vi "Cam0 AprilTag Target Package.vi"(0 "Camera Name":string="cam0") -> ()   [LabVIEW 2023]
uses:
  <vilib>/vision/Shape Detection.llb/ShapeDetectionMatchOptions.ctl
  <vilib>/vision/Pattern Matching.llb/IMAQ Match Range Setting.ctl
  <vilib>/vision/Image Controls.llb/IMAQ Image.ctl
  Camera Set Up/Event Setup Types.ctl
  <vilib>/Utility/config.llb/Write Key (String).vi
  <vilib>/Utility/config.llb/Read Key (String).vi
  <vilib>/Utility/config.llb/NI_LVConfig.lvlib
  <vilib>/vision/NI_Vision_Development_Module.lvlib
panel:
  in  "Main":enum32{"Page 1", "Page 2"}(tab)
  out "Image":T1(plugin-control)
  in  "Settings":bool
  in  "Save":bool
  in  "Tools":bool
  in  "Min Level":dbl=40.0 format="%#_13g"
  out "Fps":dbl format="%#.0f"
  in  "Target Size":dbl=6.5
  out "Distance":dbl[](array[numeric]) format="%.1f"
  out "Angle":dbl[](array[numeric]) format="%.1f"
  in  "Min Rectangle Size (pix)":dbl
  in  "Max Rectangle Size (pix)":dbl
  in  "Home":bool
  in  "Match Options":T2={"Rotation"=TRUE, "Scale"=TRUE, "Occlusion"=FALSE, "Range Settings"=[]} {"Range Settings"."Match Constraints" items=["Rotation Angle (degrees)", "Scale Factor (%)", "Occlusion (%)"]}
  in  "upper limit":sgl=1.2
  in  "lower limit":sgl=0.8
  # "Aspect Ratio"
  # "Range"
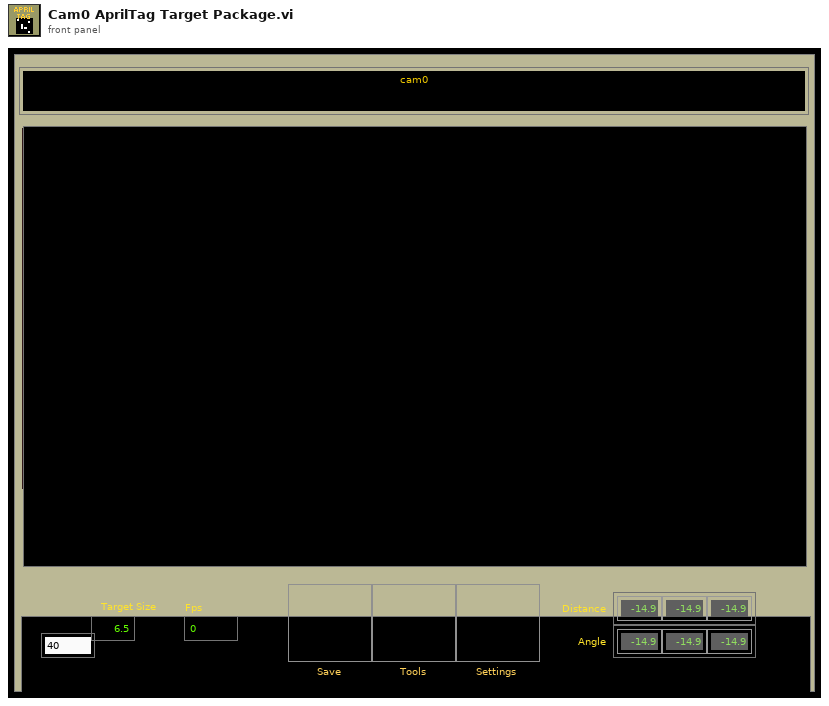
[diagram p1: front panel]
types:
  T1 = typedef "IMAQ Image.ctl" = refnum<image>
  T2 = typedef "ShapeDetectionMatchOptions.ctl" = cluster{"Rotation":bool, "Scale":bool, "Occlusion":bool, "Range Settings":T3[]}
  T3 = typedef "IMAQ Match Range Setting.ctl" = cluster{"Match Constraints":u32, "Min":dbl, "Max":dbl}
  T4 = typedef "Image Type" = u32
  T5 = cluster{"Min Width":dbl, "Max Width":dbl, "Min Height":dbl, "Max Height":dbl}
  T6 = typedef "Event Setup Types.ctl" = enum16{"Default", "Camera Loop Started", "Save Data", "Open Front Panel", "Exit"}
  T7 = cluster{"Corners":cluster{"X":sgl, "Y":sgl}[], "Angle":dbl, "Width":dbl, "Height":dbl, "Score":dbl}[]
  T8 = typedef "Target Fields.ctl" = cluster{"diameter points":cluster{"first point":cluster{"x":dbl, "y":dbl}, "projected point":cluster{"x":dbl, "y":dbl}}, "normalized center":cluster{"x":dbl, "y":dbl}, "Overall Score":dbl, "Area Score":dbl, "Moment Score":dbl, "Aspect Score":dbl, "Distance (ft)":dbl, "Upper Goal":bool}
  T9 = typedef "NI_LVConfig.lvlib/Config Data RefNum.ctl" = refnum<k1>
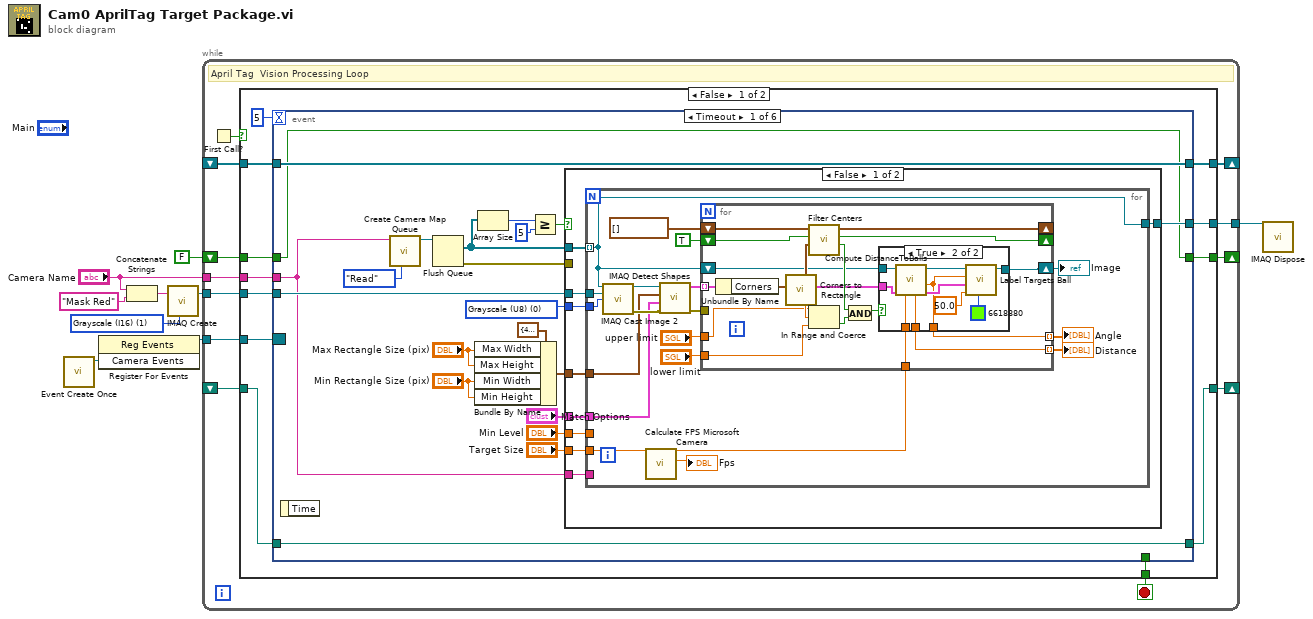
[diagram p0: block diagram]
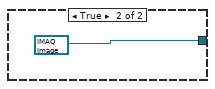
[diagram p3: hidden frame]
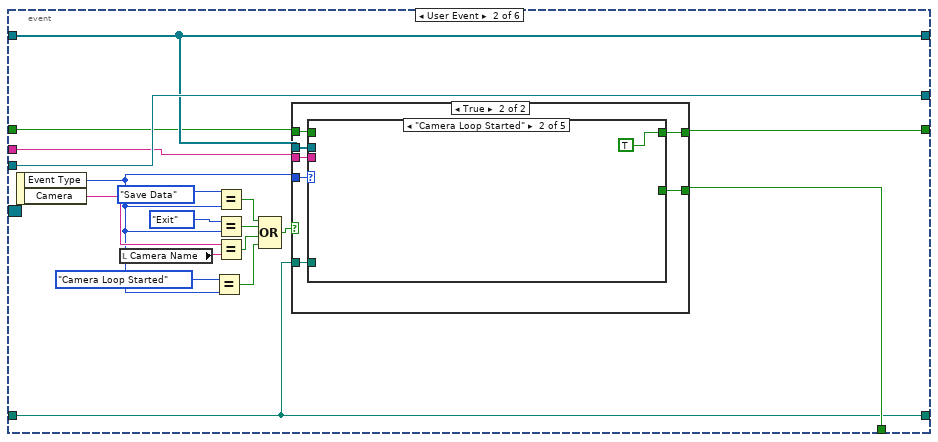
[diagram p4: hidden frame]
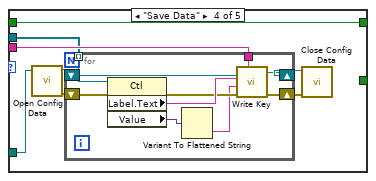
[diagram p8: hidden frame]
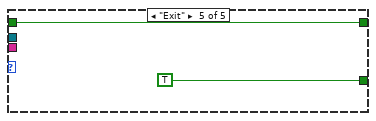
[diagram p9: hidden frame]
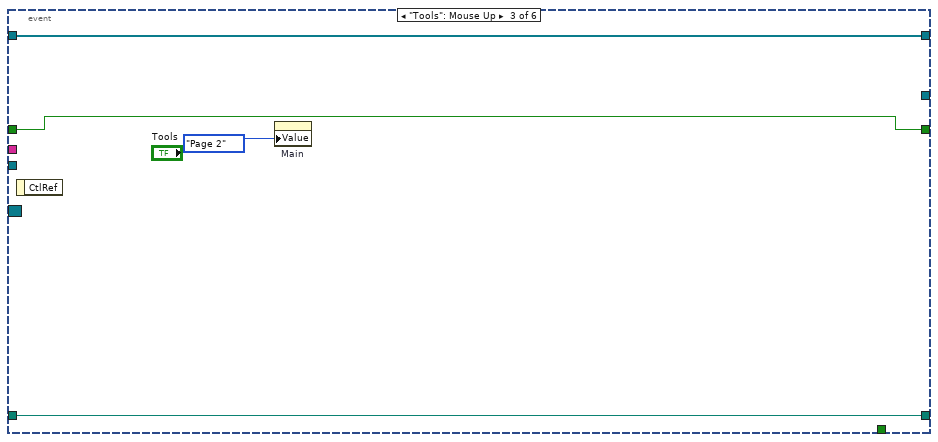
[diagram p10: hidden frame]
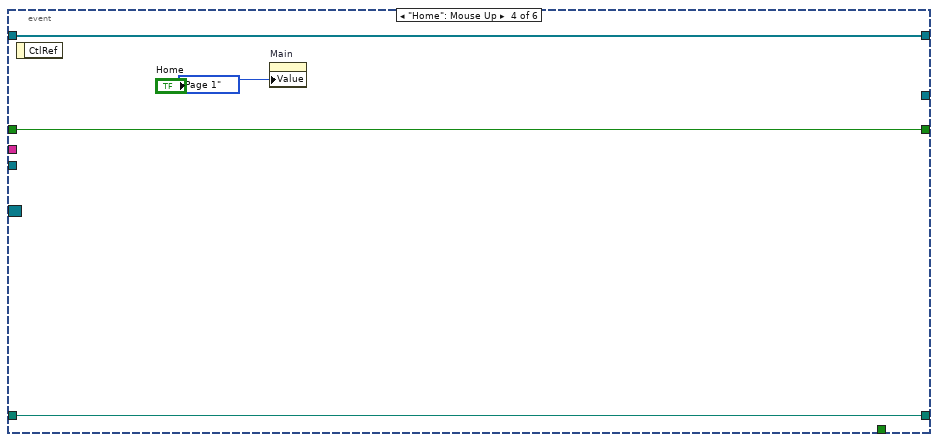
[diagram p11: hidden frame]
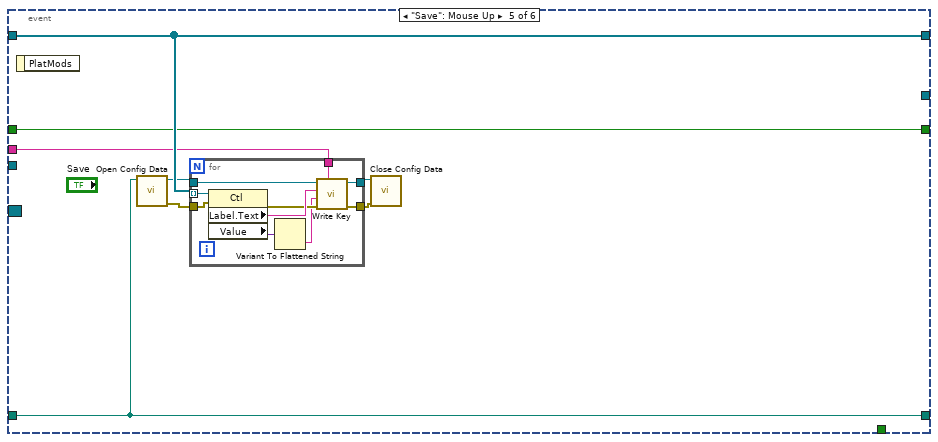
[diagram p12: hidden frame]
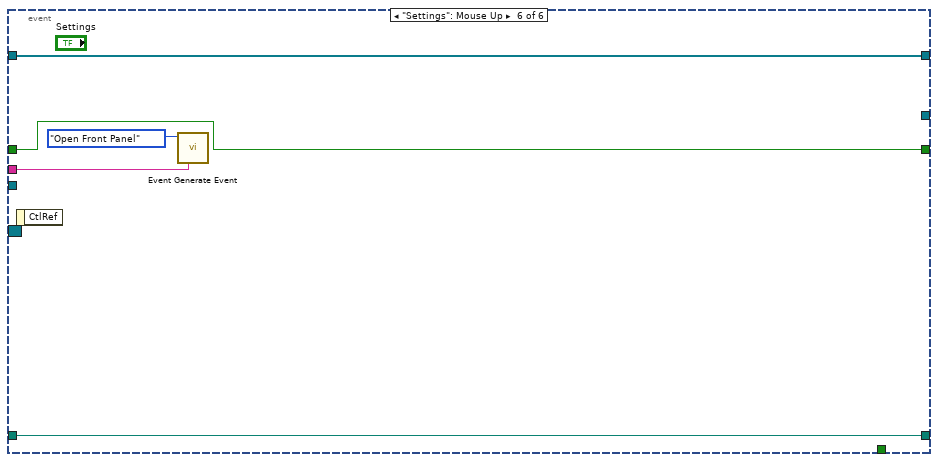
[diagram p13: hidden frame]
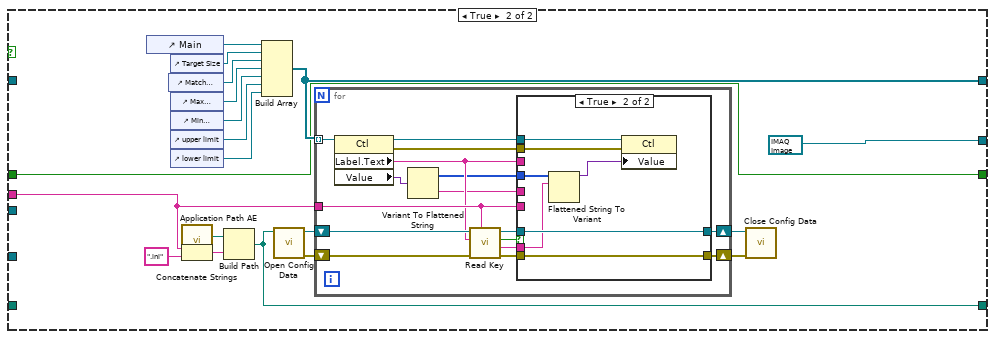
[diagram p14: hidden frame]
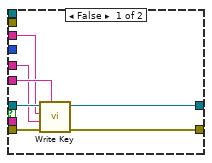
[diagram p15: hidden frame]
diagram:
  w6 = T4 1 items=["Grayscale (U8)", "Grayscale (I16)", "Grayscale (SGL)", "Complex (CSG)", "RGB (U32)", "HSL (U32)", "RGB (U64)", "Grayscale (U16)"] ("Image Type")
  n1 = call "Event Create Once.vi"() -> ("Camera Events"=w8:refnum<user-event>)  [unwired: 10 in, 1 out]
  n2 = register-events(w8) -> (reference out=w7:refnum<event-registration>)  [unwired: 2 in, 1 out]
  n3 = Concatenate Strings("Camera Name", "Mask Red" ("string")) -> (w5:string)
  n4 = call "IMAQ Create"("Image Name"=w5, "Image Type"=w6) -> ("New Image"=w9:T1)  [unwired: 2 in, 2 out]
  n5 = while {
    tunnel: w9 -> [w21]
    tunnel: [w20] -> w1
    tunnel: w7 -> [w19]
    tunnel: "Camera Name" -> [w17]
    shift-right: [w15] -> _
    shift-left: _ -> [w14]
    shift-right: [w13] -> _
    shift-left: _ -> [w12]
    shift-right: [w10] -> _
    shift-left: FALSE -> [w11]
    stop <- w18 stop-if-true
    # "April Tag  Vision Processing Loop"
    n6 = First Call?() -> (First Call?: T/F=w16:bool)
    n7 = case shown="False" w16 {
      tunnel: w21 -> [w33 _]
      tunnel: [w32 T1 refnum ("New Image")] -> w20
      tunnel: w19 -> [w31 _]
      tunnel: [w30 _] -> w18
      tunnel: w17 -> [w29 w205]
      tunnel: [w27 w201] -> w15
      tunnel: w14 -> [w28 _]
      tunnel: [w26 w204] -> w13
      tunnel: w12 -> [w24 _]
      tunnel: w11 -> [w23 w198]
      tunnel: [w22 w198] -> w10
      frame False {
        n8 = event shown="[0] Timeout" {
          selector: w31 -> [_ _ _ _ _ _]
          dyn-events: _ -> [_ _ _ _ _ _]
          timeout: 5 -> [_ _ _ _ _ _]
          tunnel: w33 -> [w53 w130 _ _ _ _]
          tunnel: [w54 w130 _ _ _ _] -> w32
          tunnel: [_ w129 _ _ _ _] -> w30
          tunnel: w29 -> [w50 w128 _ _ w173 w189]
          tunnel: w28 -> [w52 w126 w165 w169 w176 w192]
          tunnel: [w52 w126 w165 w169 w176 w192] -> w27
          tunnel: w24 -> [w51 w127 w164 w168 w177 w191]
          tunnel: [w51 w127 w164 w168 w177 w191] -> w26
          tunnel: w23 -> [w49 w117 w162 w166 w170 w188]
          tunnel: [w49 w116 w162 w166 w170 w188] -> w22
          event Timeout {
            w44 = T4 0 items=["Grayscale (U8)", "Grayscale (I16)", "Grayscale (SGL)", "Complex (CSG)", "RGB (U32)", "HSL (U32)", "RGB (U64)", "Grayscale (U16)"] ("Image Type")
            n9 = event-data() -> ()  [unwired: 1 in, 1 out]
            n10 = call "Create Camera Map Queue.vi"("Action"=enum16{"Read", "Write"}."Read", "Camera"=w50) -> ("value"=w46:refnum<queue>)  [unwired: 8 in, 1 out]
            n11 = Flush Queue(queue=w46) -> (remaining elements=w43:T1[], error out=w45:errorcluster)  [unwired: 1 in, 1 out]
            n12 = Bundle By Name(cluster=T5 {"Min Width"=40.0, "Max Width"=100.0, "Min Height"=40.0, "Max Height"=200.0} ("Rectangle Descriptor"), "Max Width"="Max Rectangle Size (pix)", "Max Height"="Max Rectangle Size (pix)", "Min Width"="Min Rectangle Size (pix)", "Min Height"="Min Rectangle Size (pix)") -> (w36:T5)
            n13 = Array Size(array=w43) -> (size(s)=w42:i32)
            n14 = Greater Or Equal?(x=w42, y=5) -> (x >= y?=w40:bool)
            n15 = case shown="False" w40 {
              tunnel: [w55 T1 refnum ("Image")] -> w54
              tunnel: w53 -> [w63 _]
              tunnel: w50 -> [w62 _]
              tunnel: "Target Size" -> [w61 _]
              tunnel: w43 -> [w60 _]
              tunnel: w45 -> [_ _]
              tunnel: w44 -> [w59 _]
              tunnel: "Min Level" -> [w58 _]
              tunnel: w36 -> [w57 _]
              tunnel: "Match Options" -> [w56 _]
              frame False {
                n16 = for {
                  tunnel: w63 -> [w81]
                  tunnel: w60 -> [w70] mode=indexing
                  tunnel: w62 -> [_]
                  tunnel: w61 -> [w69]
                  tunnel: w59 -> [w80]
                  tunnel: w58 -> [_]
                  tunnel: w57 -> [w76]
                  tunnel: w56 -> [w75]
                  tunnel: [w70] -> w55
                  n17 = call "IMAQ Cast Image 2"("Image Src"=w70, "Image Dst"=w81, "Image Type"=w80) -> ("Image Dst Out"=w78:T1, "error out"=w77:errorcluster)  [unwired: 11 in]
                  n18 = call "Calculate FPS Microsoft Camera.vi"() -> ("Fps"=→"Fps":dbl)  [unwired: 11 in]
                  n19 = call-poly "IMAQ Detect Shapes"("error in (no error)"=w77, "Match Options"=w75, "Rectangle Descriptor"=w76, "Image"=w78) -> ("error out"=w66:errorcluster, "Rectangles"=w72:T7)  [unwired: 5 in, 1 out]
                  n20 = for {
                    shift-right: [w82] -> w71
                    shift-left: w70 -> [w83]
                    shift-right: [w97] -> _
                    shift-left: cluster{"X":dbl, "Y":dbl}[] [] ("Centers 2") -> [w99]
                    shift-right: [w95] -> _
                    shift-left: TRUE -> [w96]
                    tunnel: w72 -> [w91] mode=indexing
                    tunnel: w69 -> [w88]
                    tunnel: [w87] -> w67 mode=indexing
                    tunnel: [w86] -> w68 mode=indexing
                    tunnel: w66 -> [_]
                    tunnel: "lower limit" -> [w85]
                    tunnel: "upper limit" -> [w84]
                    n21 = Unbundle By Name(w91) -> ("Corners"=w90:cluster{"X":sgl, "Y":sgl}[])
                    n22 = call "Corners to Rectangle.vi"("Corners 2"=w90) -> ("output cluster"=w89:T8, "Aspect Ratio"=w100:sgl, "Center"=w98:cluster{"X":dbl, "Y":dbl})  [unwired: 8 in]
                    n23 = call "Filter Centers.vi"("Center"=w98, "First time"=w96, "Centers"=w99) -> ("Added"=w94:bool, "First time Out"=w95:bool, "Centers 2"=w97:cluster{"X":dbl, "Y":dbl}[])  [unwired: 6 in]
                    n24 = In Range and Coerce(upper limit=w84, x=w100, lower limit=w85) -> (In Range?=w93:bool)  [unwired: 1 out]
                    n25 = And(x=w94, y=w93) -> (x .and. y?=w92:bool)
                    n26 = case shown="True" w92 {
                      tunnel: w83 -> [w101 w110]
                      tunnel: [w101 w111] -> w82
                      tunnel: w89 -> [_ w105]
                      tunnel: w88 -> [_ w104]
                      tunnel: [_ w103] -> w87
                      tunnel: [_ w102] -> w86
                      frame False {
                      }
                      frame True {
                        n27 = call "Compute DistanceToBalls.vi"("Target Width (in)"=w104, "results"=w105, "Image Src"=w110) -> ("results out"=w106:T8, "Off Angle"=w102:dbl, "Image Dst Out"=w108:T1, "Distance"=w103:dbl)  [unwired: 4 in, 1 out]
                        n28 = call "Label Targets Ball.vi"("Color"=u32 6618880, "Score Threshold"=50.0, "results"=w106, "Angle"=w102, "Image in"=w108) -> ("Image out"=w111:T1)  [unwired: 6 in]
                      }
                    }
                  }
                  "Image" <- w71
                  "Angle" <- w68
                  "Distance" <- w67
                }
              }
              frame True {
              }
            }
          }
          event User Event {
            n29 = event-data() -> ("Event Type"=w115:T6, "Camera"=w120:string)  [unwired: 1 in]
            n30 = local read "Camera Name"() -> (w121:string)
            n31 = Equal?(x=Event_Setup_Types."Camera Loop Started", y=w115) -> (x = y?=w113:bool)
            n32 = Equal?(x=Event_Setup_Types."Save Data", y=w115) -> (x = y?=w122:bool)
            n33 = Equal?(x=Event_Setup_Types."Exit", y=w115) -> (x = y?=w124:bool)
            n34 = Equal?(x=w120, y=w121) -> (x = y?=w119:bool)
            n35 = Compound Arithmetic op=OR(w122, w124, w119, w113) -> (w118:bool)
            n36 = case shown="True" w118 {
              tunnel: w115 -> [_ w138]
              tunnel: [_ w137] -> w129
              tunnel: w128 -> [_ w136]
              tunnel: w127 -> [_ w135]
              tunnel: w126 -> [_ w134]
              tunnel: w117 -> [w131 w133]
              tunnel: [w131 w132] -> w116
              frame False {
              }
              frame True {
                n37 = case shown="\"Camera Loop Started\"" w138 {
                  tunnel: [_ _ _ _ TRUE] -> w137
                  tunnel: w136 -> [_ _ _ w145 _]
                  tunnel: w135 -> [_ _ _ w144 _]
                  tunnel: w134 -> [_ _ _ w143 _]
                  tunnel: w133 -> [w139 _ w141 w142 w160]
                  tunnel: [w139 TRUE w141 w142 w160] -> w132
                  frame "Default" {
                  }
                  frame "Camera Loop Started" {
                  }
                  frame "Open Front Panel" {
                  }
                  frame "Save Data" {
                    n38 = call <vilib>:"Open Config Data.vi"("configuration file path"=w144) -> ("error out"=w146:errorcluster, "refnum"=w149:T9)  [unwired: 8 in, 1 out]
                    n39 = for {
                      tunnel: w145 -> [w155]
                      tunnel: w143 -> [w154] mode=indexing
                      shift-right: [w158] -> w148
                      shift-left: w149 -> [w159]
                      shift-right: [w157] -> w147
                      shift-left: w146 -> [w156]
                      n40 = property class="Ctl"(reference=w154, error in=w156) -> (error out=w151:errorcluster, "Label.Text"=w153:string, "Value"=w152:variant)  [unwired: 1 out]
                      n41 = Variant To Flattened String(Variant=w152) -> (data string=w150:string)  [unwired: 1 out]
                      n42 = call-poly <vilib>:"Write Key.vi"("section"=w155, "error in (no error)"=w151, "value"=w150, "key"=w153, "refnum"=w159) -> ("error out"=w157:errorcluster, "refnum out"=w158:T9)  [unwired: 4 in, 1 out]
                    }
                    n43 = call <vilib>:"Close Config Data.vi"("error in (no error)"=w147, "refnum"=w148) -> ()  [unwired: 8 in, 2 out]
                  }
                  frame "Exit" {
                  }
                }
              }
            }
          }
          event "Tools": Mouse Up {
            n44 = event-data() -> ()  [unwired: 1 in, 1 out]
            n45 = property on="Main" class="TabCtl (strict)"("Value"=enum32{"Page 1", "Page 2"}."Page 2" ("Main")) -> ()  [unwired: 2 in, 2 out]
          }
          event "Home": Mouse Up {
            n46 = event-data() -> ()  [unwired: 1 in, 1 out]
            n47 = property on="Main" class="TabCtl (strict)"("Value"=enum32{"Page 1", "Page 2"}."Page 1" ("Main")) -> ()  [unwired: 2 in, 2 out]
          }
          event "Save": Mouse Up {
            n48 = event-data() -> ()  [unwired: 1 in, 1 out]
            n49 = call <vilib>:"Open Config Data.vi"("configuration file path"=w177) -> ("error out"=w174:errorcluster, "refnum"=w175:T9)  [unwired: 8 in, 1 out]
            n50 = for {
              tunnel: w176 -> [w187] mode=indexing
              tunnel: w175 -> [w186]
              tunnel: w174 -> [w185]
              tunnel: w173 -> [w181]
              tunnel: [w179] -> w172
              tunnel: [w178] -> w171
              n51 = property class="Ctl"(reference=w187, error in=w185) -> (error out=w182:errorcluster, "Label.Text"=w184:string, "Value"=w183:variant)  [unwired: 1 out]
              n52 = Variant To Flattened String(Variant=w183) -> (data string=w180:string)  [unwired: 1 out]
              n53 = call-poly <vilib>:"Write Key.vi"("section"=w181, "error in (no error)"=w182, "value"=w180, "key"=w184, "refnum"=w186) -> ("error out"=w179:errorcluster, "refnum out"=w178:T9)  [unwired: 4 in, 1 out]
            }
            n54 = call <vilib>:"Close Config Data.vi"("error in (no error)"=w172, "refnum"=w171) -> ()  [unwired: 8 in, 2 out]
          }
          event "Settings": Mouse Up {
            n55 = event-data() -> ()  [unwired: 1 in, 1 out]
            n56 = call "Event Generate Event.vi"("Camera Name"=w189, "Event Type"=Event_Setup_Types."Open Front Panel") -> ()  [unwired: 10 in]
          }
        }
      }
      frame True {
        n57 = control-ref of="Main"() -> (w200:refnum<vi>)
        n58 = control-ref of="Match Options"() -> (w197:refnum<vi>)
        n59 = control-ref of="Target Size"() -> (w199:refnum<vi>)
        n60 = control-ref of="Max Rectangle Size (pix)"() -> (w196:refnum<vi>)
        n61 = control-ref of="Min Rectangle Size (pix)"() -> (w195:refnum<vi>)
        n62 = control-ref of="upper limit"() -> (w194:refnum<vi>)
        n63 = control-ref of="lower limit"() -> (w193:refnum<vi>)
        n64 = call "Application Path AE.vi"() -> ("Application Path out"=w202:path)  [unwired: 11 in]
        n65 = Concatenate Strings(w205, ".ini" ("name or relative path")) -> (w210:string)
        n66 = Build Path(base path=w202, name or relative path=w210) -> (appended path=w204:path)
        n67 = Build Array(w200, w199, w197, w196, w195, w194, w193) -> (w201:refnum<vi>[])
        n68 = call <vilib>:"Open Config Data.vi"("configuration file path"=w204) -> ("error out"=w203:errorcluster, "refnum"=w209:T9)  [unwired: 8 in, 1 out]
        n69 = for {
          tunnel: w205 -> [w224]
          tunnel: w201 -> [w214] mode=indexing
          shift-right: [w226] -> w208
          shift-left: w209 -> [w227]
          shift-right: [w225] -> w207
          shift-left: w203 -> [w223]
          n70 = property class="Ctl"(reference=w214) -> (reference out=w220:refnum<vi>, error out=w219:errorcluster, "Label.Text"=w217:string, "Value"=w213:variant)  [unwired: 1 in]
          n71 = Variant To Flattened String(Variant=w213) -> (data string=w215:string, 1:w212:i16[])
          n72 = call-poly <vilib>:"Read Key.vi"("section"=w224, "error in (no error)"=w223, "key"=w217, "refnum"=w227) -> ("error out"=w216:errorcluster, "value"=w221:string, "found?"=w222:bool, "refnum out"=w218:T9)  [unwired: 4 in]
          n73 = case shown="True" w222 {
            tunnel: w221 -> [_ w236]
            tunnel: w220 -> [_ w241]
            tunnel: w219 -> [_ w240]
            tunnel: w218 -> [w234 w239]
            tunnel: w224 -> [w233 _]
            tunnel: w217 -> [w232 _]
            tunnel: [w231 w239] -> w226
            tunnel: w216 -> [w230 w238]
            tunnel: [w229 w238] -> w225
            tunnel: w215 -> [w228 _]
            tunnel: w212 -> [_ w235]
            frame False {
              n74 = call-poly <vilib>:"Write Key.vi"("section"=w233, "error in (no error)"=w230, "value"=w228, "key"=w232, "refnum"=w234) -> ("error out"=w229:errorcluster, "refnum out"=w231:T9)  [unwired: 4 in, 1 out]
            }
            frame True {
              n75 = Flattened String To Variant(6:w236, 7:w235) -> (3:w237:variant)  [unwired: 1 in, 1 out]
              n76 = property class="Ctl"(reference=w241, error in=w240, "Value"=w237) -> ()  [unwired: 2 out]
            }
          }
        }
        n77 = call <vilib>:"Close Config Data.vi"("error in (no error)"=w207, "refnum"=w208) -> ()  [unwired: 8 in, 2 out]
      }
    }
  }
  n78 = call "IMAQ Dispose"("Image"=w1) -> ()  [unwired: 5 in, 1 out]
